vi "FTW-ActorContext-Construct.vi"(5 "Address (blank for Local Application Context)":string, 7 "Port":u16=3363, 9 "Timeout":i32=10000, 11 "error in":errorcluster) -> (4 "FTW Actor Context":refnum<class "FTW-Actor-Context.lvclass">, 15 "error out":errorcluster)   [LabVIEW 2015, in "FTW-Actor-Context.lvclass"]
uses:
  FTW-Actor-Context.lvclass
  FTW-Actor-Context.lvclass/FTW-Actor-Context.ctl
panel:
  # "Inputs"
  # "Outputs"
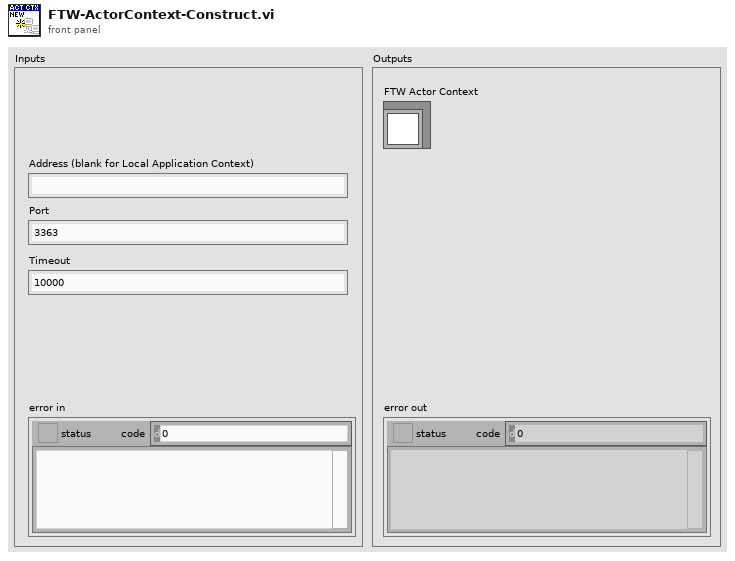
[diagram p1: front panel]
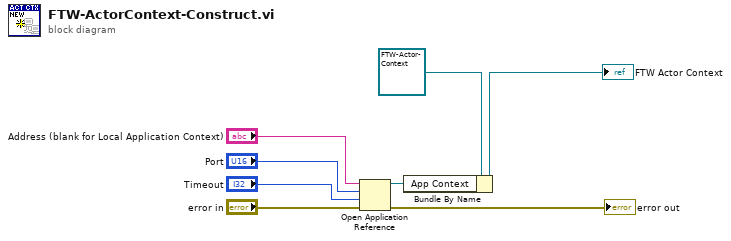
[diagram p0: block diagram]
diagram:
  n1 = Open Application Reference(8:"error in", 9:"Timeout", 10:"Port", 11:"Address (blank for Local Application Context)") -> (0:→"error out":errorcluster, 3:w6:refnum<vi>)
  n2 = Bundle By Name(cluster=refnum<class "FTW-Actor-Context.lvclass"> refnum ("FTW Actor Context"), "App Context"=w6) -> (→"FTW Actor Context":refnum<class "FTW-Actor-Context.lvclass">)
